vi "Stop Collecting and Return Data.vi"(8 "error in (no error)":errorcluster) -> (0 "error out":errorcluster, 1 "data value reference":refnum<data-value>, 2 "Array Size":u32, 3 "Success":bool, 5 "CD_Status":i32)   [LabVIEW 2015, in "Tool Module.lvlib"]
uses:
  Tool Module.lvlib
  Collect Data Mgr/Collect Data Mgr.lvlib
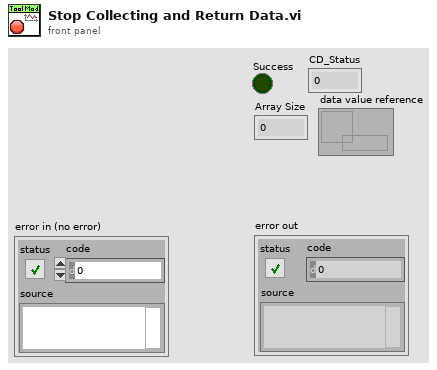
[diagram p1: front panel]
types:
  T1 = typedef "Collect Data Mgr.lvlib/Stop Collect (Reply Payload)--cluster.ctl" = cluster{"Success":bool, "CD_Status":i32, "Array Size":u32, "data value reference":refnum<data-value>}
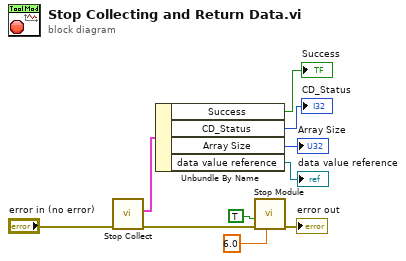
[diagram p0: block diagram]
diagram:
  n1 = call "Stop Collect.vi"("error in (no error)"="error in (no error)") -> ("error out"=w1:errorcluster, "Reply Payload"=w9:T1)  [unwired: 8 in, 1 out]
  n2 = Unbundle By Name(w9) -> ("Success"=→"Success":bool, "CD_Status"=→"CD_Status":i32, "Array Size"=→"Array Size":u32, "data value reference"=→"data value reference":refnum<data-value>)
  n3 = call "Stop Module.vi"("Timeout to Wait for Stop (s) (-1: no timeout)"=6.0, "error in (no error)"=w1, "Wait for Module to Stop? (F)"=TRUE) -> ("error out"=→"error out":errorcluster)  [unwired: 8 in]
